vi "testIRdet3.vi"(8 "error in (no error)":errorcluster, 11 "y":dbl) -> (0 "error out":errorcluster, 1 "公分":dbl(slide) scale=0.0..200.0, 2 "差值":dbl[](array[numeric]), 3 "power":dbl[](array[numeric]))   [LabVIEW 2019]
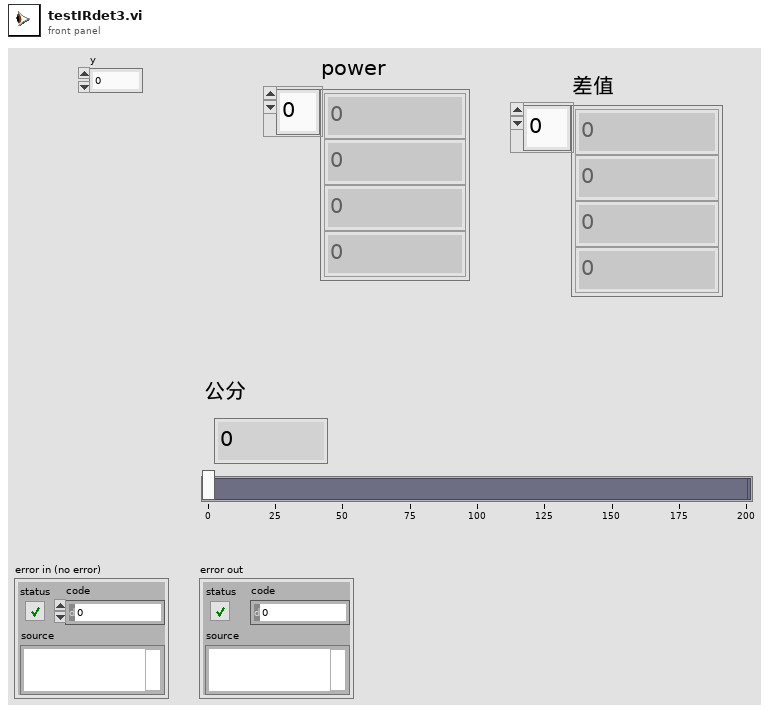
[diagram p1: front panel]
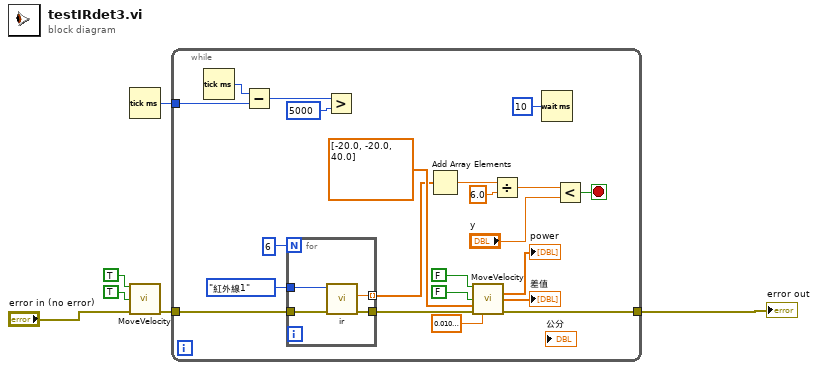
[diagram p0: block diagram]
diagram:
  n1 = Tick Count (ms)() -> (millisecond timer value=w1:u32)
  n2 = call "MoveVelocity.vi"("reinitialize? (F)"=TRUE, "EncRst"=TRUE, "error in (no error)"="error in (no error)") -> ("error out"=w3:errorcluster)  [unwired: 9 in, 3 out]
  n3 = while {
    tunnel: w1 -> [w27]
    tunnel: [w23] -> w2
    tunnel: w3 -> [w15]
    stop <- w17 stop-if-true
    n4 = Tick Count (ms)() -> (millisecond timer value=w28:u32)
    n5 = Subtract(x=w28, y=w27) -> (x-y=w26:u32)
    n6 = for {
      N: 6 -> [_]
      tunnel: w15 -> [w32]
      tunnel: enum16{"請選擇紅外線", "紅外線1", "紅外線2", "紅外線3", "紅外線4"}."紅外線1" ("選擇紅外線") -> [w31]
      tunnel: [w30] -> w13
      tunnel: [w29] -> w12 mode=indexing
      n7 = call "ir.vi"("error in (no error)"=w32, "選擇紅外線"=w31) -> ("error out"=w30:errorcluster, "公分"=w29:dbl)  [unwired: 8 in]
    }
    n8 = Greater?(x=w26, y=u32 5000) -> ()  [unwired: 1 out]
    n9 = Add Array Elements(numeric array=w12) -> (sum=w11:dbl)
    n10 = call "MoveVelocity.vi"("reinitialize? (F)"=FALSE, "EncRst"=FALSE, "OBJ"=dbl[] [-20.0, -20.0, 40.0], "error in (no error)"=w13, "dt (s)"=0.010000000000000002) -> ("power"=→"power":dbl[], "差值"=→"差值":dbl[], "error out"=w23:errorcluster)  [unwired: 7 in, 1 out]
    n11 = Divide(x=w11, y=6.0) -> (x/y=w9:dbl)
    n12 = Wait (ms)(milliseconds to wait=u32 10) -> ()  [unwired: 1 out]
    n13 = Less?(x=w9, y="y") -> (x < y?=w17:bool)
  }
  "error out" <- w2
